vi "USB-4000 MultiAi.vi"() -> ()   [LabVIEW 2016]
panel:
  in  "Range":sgl=10.0
  out "error out":errorcluster caption="错误输出"
  in  "停止":bool
  out "波形图":cluster{dbl, dbl, sgl[][]}(graph)
  in  "读取通道选择":T1={"CH 0"=TRUE, "CH 1"=TRUE, "CH 2"=TRUE, "CH 3"=TRUE, "CH 4"=TRUE, "CH 5"=TRUE, "CH 6"=TRUE, "CH 7"=TRUE, "CH 8"=FALSE, "CH 9"=FALSE, "CH 10"=FALSE, "CH 11"=FALSE, "CH 12"=FALSE, "CH 13"=FALSE, "CH 14"=FALSE, "CH 15"=FALSE}
  in  "Num":u32=50000 caption="每通道读取点数"
  in  "SampleRate":u32=500000 caption="SampleRate (pts/s)"
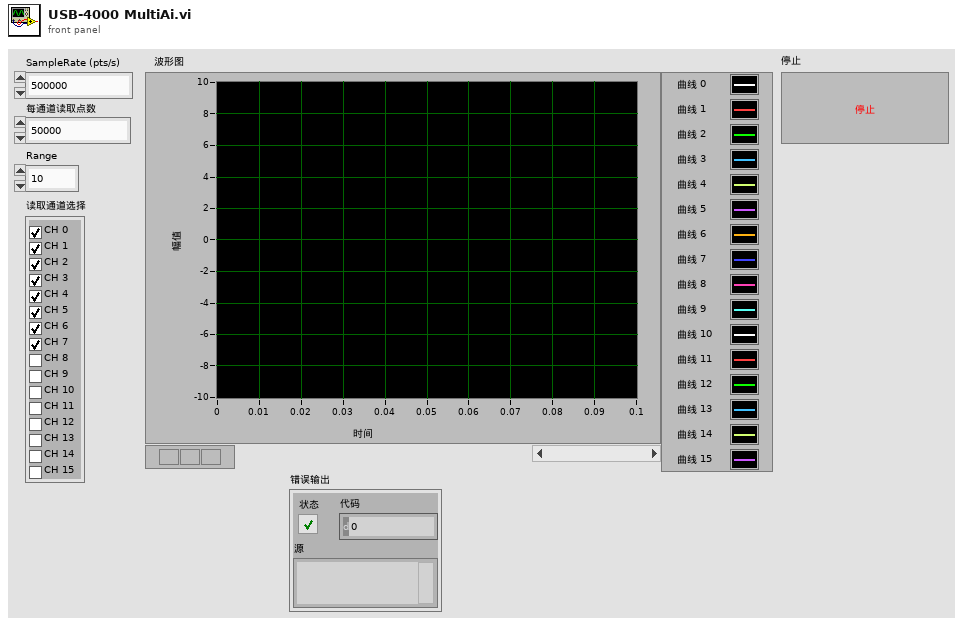
[diagram p1: front panel]
types:
  T1 = cluster{"CH 0":bool, "CH 1":bool, "CH 2":bool, "CH 3":bool, "CH 4":bool, "CH 5":bool, "CH 6":bool, "CH 7":bool, "CH 8":bool, "CH 9":bool, "CH 10":bool, "CH 11":bool, "CH 12":bool, "CH 13":bool, "CH 14":bool, "CH 15":bool}
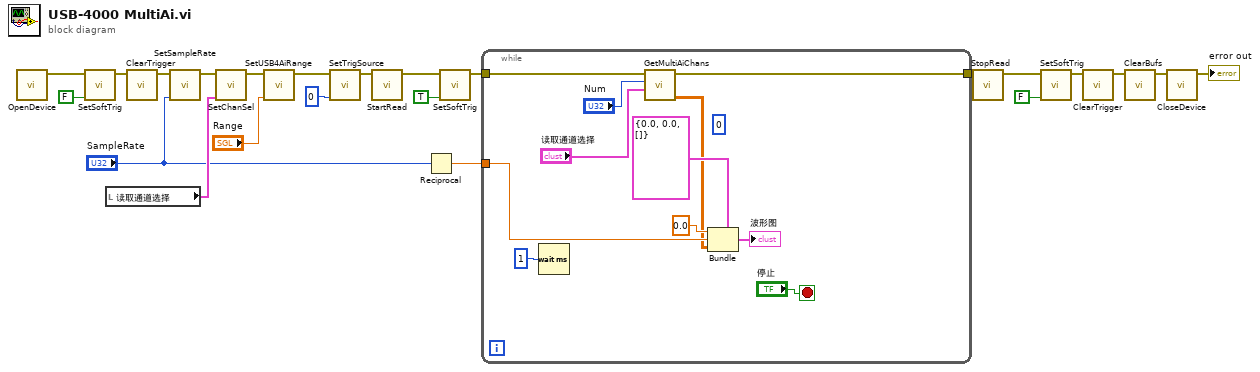
[diagram p0: block diagram]
diagram:
  n1 = call "OpenDevice.vi"() -> ("error out"=w4:errorcluster)  [unwired: 11 in]
  n2 = call "SetSoftTrig.vi"("SoftTrig"=FALSE, "error in"=w4) -> ("error out"=w7:errorcluster)  [unwired: 9 in]
  n3 = local read "读取通道选择"() -> (w14:T1)
  n4 = call "ClearTrigger.vi"("错误输入（无错误）"=w7) -> ("错误输出"=w5:errorcluster)  [unwired: 10 in]
  n5 = call "SetSampleRate.vi"("SampleRate"="SampleRate", "error in"=w5) -> ("error out"=w12:errorcluster)  [unwired: 9 in]
  n6 = call "SetChanSel.vi"("读取通道选择"=w14, "错误输入"=w12) -> ("错误输出"=w15:errorcluster)  [unwired: 9 in]
  n7 = call "SetUSB4AiRange.vi"("Range"="Range", "error in"=w15) -> ("error out"=w11:errorcluster)  [unwired: 9 in]
  n8 = call "SetTrigSource.vi"("TrigSource"=u8 0, "error in"=w11) -> ("error out"=w1:errorcluster)  [unwired: 9 in]
  n9 = call "StartRead.vi"("error in"=w1) -> ("error out"=w2:errorcluster)  [unwired: 10 in]
  n10 = Reciprocal(x="SampleRate") -> (1/x=w18:dbl)
  n11 = call "SetSoftTrig.vi"("SoftTrig"=TRUE, "error in"=w2) -> ("error out"=w3:errorcluster)  [unwired: 9 in]
  n12 = while {
    tunnel: w3 -> [w34]
    tunnel: w18 -> [w27]
    tunnel: [w25] -> w17
    stop <- "停止" stop-if-true
    (unwired) 0 ("索引 (行)")
    n13 = Wait (ms)(milliseconds to wait=u32 1 ("等待时间（毫秒）")) -> ()  [unwired: 1 out]
    n14 = call "GetMultiAiChans.vi"("ChansSel"="读取通道选择", "Num"="Num", "error in"=w34) -> ("Data"=w24:sgl[][], "error out"=w25:errorcluster)  [unwired: 7 in]
    n15 = Bundle(cluster=cluster{dbl, dbl, sgl[][]} {0.0, 0.0, []}, 0.0, w27, w24) -> (→"波形图":cluster{dbl, dbl, sgl[][]})
  }
  n16 = call "StopRead.vi"("error in"=w17) -> ("error out"=w23:errorcluster)  [unwired: 10 in]
  n17 = call "SetSoftTrig.vi"("SoftTrig"=FALSE, "error in"=w23) -> ("error out"=w8:errorcluster)  [unwired: 9 in]
  n18 = call "ClearTrigger.vi"("错误输入（无错误）"=w8) -> ("错误输出"=w9:errorcluster)  [unwired: 10 in]
  n19 = call "ClearBufs.vi"("error in"=w9) -> ("error out"=w20:errorcluster)  [unwired: 10 in]
  n20 = call "CloseDevice.vi"("error in"=w20) -> ("error out"=→"error out":errorcluster)  [unwired: 10 in]
